vi "BRig_RT__Case_Exp__State_ENLPre__v3.vi"(6 "input_ENL2":bool, 7 "input_I_lick":bool, 9 "input_dataTrial":u16[][](array[numeric]), 11 "input_dataCurrent":u16[](array[numeric])) -> (1 "output_dataTrial":u16[][](array[numeric]), 3 "output_dataCurrent":u16[](array[numeric]), 5 "output_state":T1)   [LabVIEW 2014]
uses:
  myRIO_BRig_RT__Case_Exp_stateList.ctl
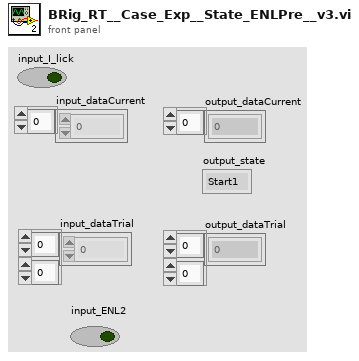
[diagram p1: front panel]
types:
  T1 = typedef "myRIO_BRig_RT__Case_Exp_stateList.ctl" = enum16{"Start1", "Start2", "Start3", "saveSettings1", "saveSettings2", "saveSettings3", "saveSettings4", "saveSettings_LC_ENL_l1", "saveSettings_LC_ENL_l2", "saveSettings_LC_Cue_l1", "saveSettings_LC_Cue_l2", "saveSettings6_LC_l1_Other", "SaveSettings6_LC_l2_Other", "setSettings_Audio", "setSettings_Laser", "initBlock_pre", "initBlock", "initBlock2", "initBlock_post", "initTrial_pre", "initTrial", "initTrial2", "initTrial3", "initTrial4", "initTrial_LC_ENL1", "initTrial_LC_Cue1", "initTrial_LC_Cue1_2", "initTrial_LC_Sel", "initTrial_post", "ENL1_pre", "ENL1", "ENL1_post", "ENL1Penalty_pre", "ENL1Penalty", "ENL2_pre", "ENL2", "ENL2Penalty_pre", "ENL2Penalty", "Cue1_pre", "Cue1", "Cue1_post", "Cue1Penalty_pre", "Cue1Penalty", "Cue2_pre", "Cue2", "Cue2Penalty_pre", "Cue2Penalty", "Selection_pre", "Selection", "Select_post", "SelectReward_pre", "SelectReward", "SelectRewardPost_pre", "SelectRewardPost", "SelectWrong_pre", "SelectWrong", "SelectWrong_post", "SelectTimeout_pre", "SelectTimeout", "SelectTimeout_post", "endTrial_pre", "endTrial1", "endTrial2", "endTrial3", "endTrial_post", "endBlock_pre", "endBlock", "endBlock_post", "endExp", "commConnect", "commUpload_pre", "commUpload_dataBlock", "commUpload_dataCurrent", "commUpload_dataExp", "commUpload_dataLC", "commUpload_dataTrial", "commUpload_post", "saveData_pre", "saveData_dataBlock", "saveData_dataCurrent", "saveData_dataExp", "saveData_dataLC", "saveData_dataTrial", "saveData_post", "empty_endBlock1", "empty_endBlock2", "empty_endTrial1", "empty_endTrial2", "empty_endTrial3", "empty_endTrial4", "empty_endTrial5", "dummyState", "dummyState_endBlock", "FreeReward_pre", "FreeReward", "FreeRewardPost_pre", "FreeRewardPost"}
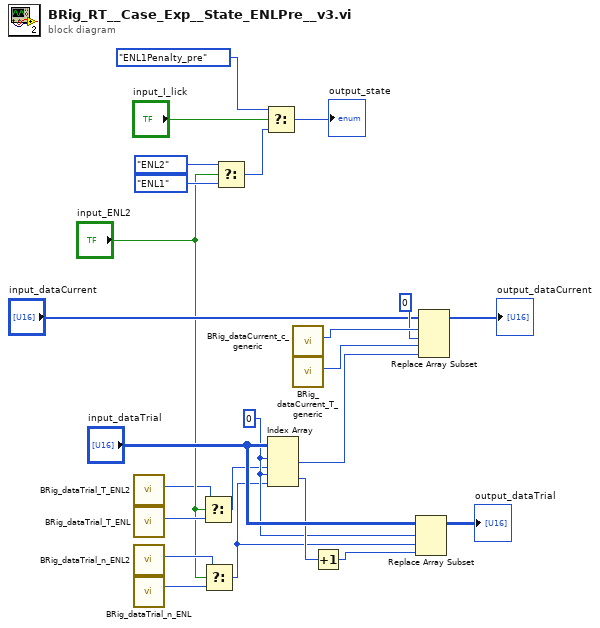
[diagram p0: block diagram]
diagram:
  w12 = 0
  n1 = call "BRig_dataTrial_T_ENL2.vi"() -> ("output_T_ENL2"=w1:i32)  [unwired: 11 in]
  n2 = call "BRig_dataTrial_T_ENL.vi"() -> ("output_T_ENL"=w4:i32)  [unwired: 11 in]
  n3 = call "BRig_dataTrial_n_ENL2.vi"() -> ("output_ENL2_n"=w7:i32)  [unwired: 11 in]
  n4 = call "BRig_dataTrial_n_ENL.vi"() -> ("output_ENL_n"=w6:i32)  [unwired: 11 in]
  n5 = Select(t=w1, s="input_ENL2", f=w4) -> (s? t:f=w3:i32)
  n6 = Select(t=w7, s="input_ENL2", f=w6) -> (s? t:f=w5:i32)
  n7 = Select(t=myRIO_BRig_RT__Case_Exp_stateList."ENL2" ("Enum"), s="input_ENL2", f=myRIO_BRig_RT__Case_Exp_stateList."ENL1" ("Enum")) -> (s? t:f=w8:T1)
  n8 = Select(t=myRIO_BRig_RT__Case_Exp_stateList."ENL1Penalty_pre" ("Enum"), s="input_I_lick", f=w8) -> (s? t:f=→"output_state":T1)
  n9 = Index Array(array="input_dataTrial", index (row) #1=w12, index (col) #1=w3, index (row) #2=w12, index (col) #2=w5) -> (element #1=w22:u16, element #2=w15:u16)
  n10 = call "BRig_dataCurrent_c_generic.vi"() -> ("output_count_generic"=w24:i32)  [unwired: 11 in]
  n11 = call "BRig_dataCurrent_T_generic.vi"() -> ("output_T_generic"=w23:i32)  [unwired: 11 in]
  n12 = Increment(x=w15) -> (x+1=w14:u16)
  n13 = Replace Array Subset(array="input_dataTrial", new element=w14, index (row)=w12, index (col)=w5) -> (→"output_dataTrial":u16[][])
  n14 = Replace Array Subset(array="input_dataCurrent", new element #1=u16 0 ("new element/subarray"), index #1=w24, new element #2=w22, index #2=w23) -> (→"output_dataCurrent":u16[])
